vi "picoquant_close_dset.vi"(8 "error in (no error)":errorcluster, 11 "picoharp in":refnum<class "picoharp.lvclass">) -> (0 "error out":errorcluster, 3 "picoharp out":refnum<class "picoharp.lvclass">)   [LabVIEW 2015, in "picoharp.lvclass"]
uses:
  picoharp.lvclass
  picoharp.lvclass/picoharp.ctl
  Data Logger Class/data_logger.lvclass
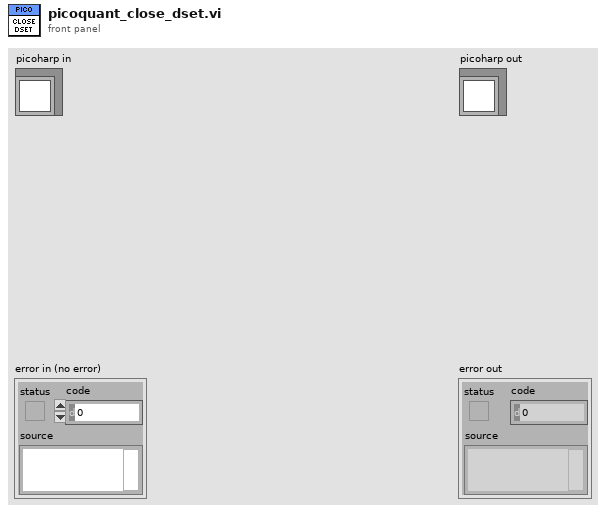
[diagram p1: front panel]
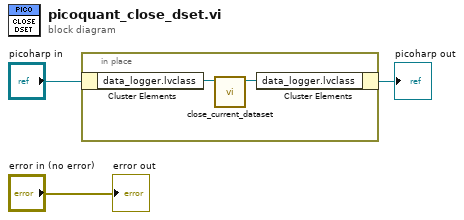
[diagram p0: block diagram]
diagram:
  n1 = in-place {
    n2 = in-place-cluster #1("picoharp in") -> ("data_logger.lvclass"=w5:refnum<class "data_logger.lvclass">)
    n3 = call-dynamic "close_current_dataset.vi"("data_logger in"=w5) -> ("data_logger out"=w4:refnum<class "data_logger.lvclass">)  [unwired: 9 in, 1 out]
    n4 = in-place-cluster #1("data_logger.lvclass"=w4) -> (→"picoharp out":refnum<class "picoharp.lvclass">)
  }
  "error out" <- "error in (no error)"
